vi "IO_MFA_DIN_Read_DigitalInput_DriveEnableSwitch.vi"() -> (3 "DriveEnableSwitch":bool)   [LabVIEW 2011]
panel:
  out "error DriveEnableSwitch":errorcluster
  out "AAABuild":i32
  in  "MintController":refnum<k7>(container)
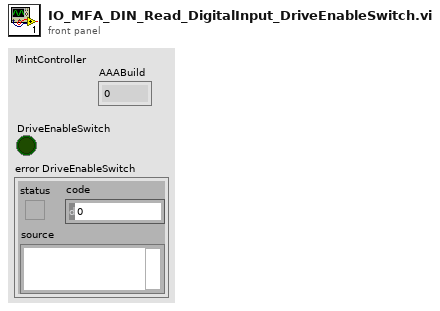
[diagram p1: front panel]
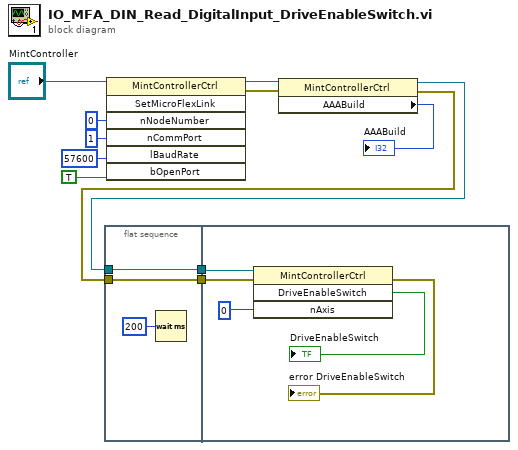
[diagram p0: block diagram]
diagram:
  n1 = flat-sequence {
    tunnel: w3 -> [w14]
    tunnel: w4 -> [w15]
    tunnel: [w15] -> w2
    tunnel: [w14] -> w1
    tunnel: w2 -> [w19]
    tunnel: w1 -> [w18]
    frame #0 {
      n2 = Wait (ms)(milliseconds to wait=u32 200) -> ()  [unwired: 1 out]
    }
    frame #1 {
      n3 = invoke class="MintControllerCtrl" method="DriveEnableSwitch"(reference=w18, error in=w19, "nAxis"=i16 0) -> (error out=→"error DriveEnableSwitch":errorcluster, "DriveEnableSwitch"=→"DriveEnableSwitch":bool)  [unwired: 1 in, 2 out]
    }
  }
  n4 = invoke class="MintControllerCtrl" method="SetMicroFlexLink"(reference="MintController", "nNodeNumber"=i16 0, "nCommPort"=i16 1, "lBaudRate"=57600, "bOpenPort"=TRUE) -> (reference out=w12:refnum<k7>, error out=w6:errorcluster)  [unwired: 2 in, 5 out]
  n5 = property class="MintControllerCtrl"(reference=w12, error in=w6) -> (reference out=w3:refnum<k7>, error out=w4:errorcluster, "AAABuild"=→"AAABuild":i32)
